vi "Auton_Selector.vi"(11 "Auton Name In":string) -> (3 "Auton Steps":T1[](array[typedef]))   [LabVIEW 2019]
uses:
  Drive/Drive Command Typedef.ctl
  Drive/Drive Mode Typedef.ctl
  Shoot/Shooter Command Type Def.ctl
  Shoot/Shooter Mode Type Def.ctl
  Intake/Intake Command Type Def.ctl
  Intake/Intake Mode Type Def.ctl
  <vilib>/Rock Robotics/WPI/Solenoid/WPI_SolenoidValue.ctl
  Auton Subsystems Steps Typedef.ctl
panel:
  in  "Possible autons":T9(array[cluster])
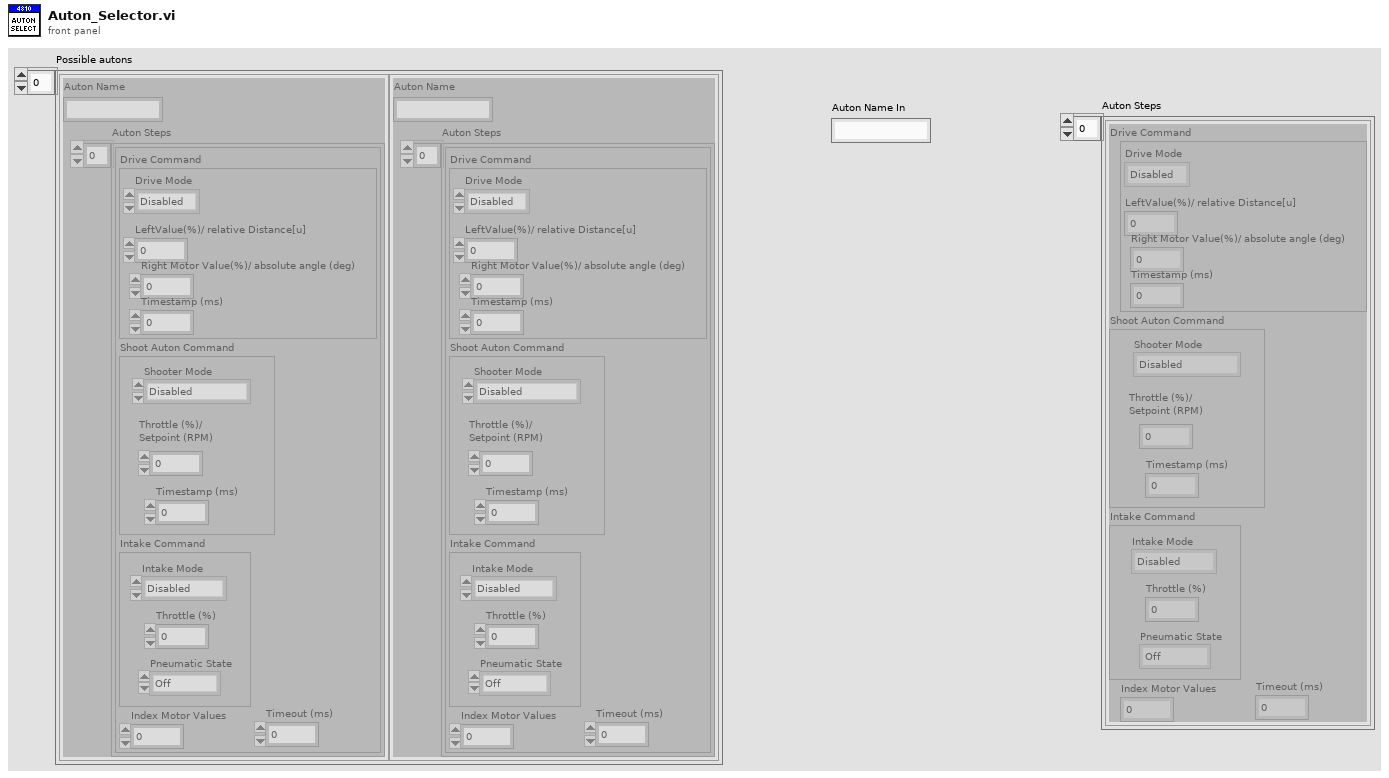
[diagram p1: front panel]
types:
  T1 = typedef "Auton Subsystems Steps Typedef.ctl" = cluster{"Drive Command":T2, "Shoot Auton Command":T4, "Intake Command":T6, "Index Motor Values":dbl, "Timeout (ms)":dbl}
  T2 = typedef "Drive Command Typedef.ctl" = cluster{"Drive Mode":T3, "LeftValue(%)/ relative Distance[u]":dbl, "Right Motor Value(%)/ absolute angle (deg)":dbl, "Timestamp (ms)":dbl}
  T3 = typedef "Drive Mode Typedef.ctl" = enum16{"Disabled", "Auto-align", "Drive Distance", "Turn to angle", "Driver"}
  T4 = typedef "Shooter Command Type Def.ctl" = cluster{"Shooter Mode":T5, "Throttle (%)/ \nSetpoint (RPM)":dbl, "Timestamp (ms)":dbl}
  T5 = typedef "Shooter Mode Type Def.ctl" = enum16{"Disabled", "Raw Throttle", "Velocity Control"}
  T6 = typedef "Intake Command Type Def.ctl" = cluster{"Intake Mode":T7, "Throttle (%)":dbl, "Pneumatic State":T8}
  T7 = typedef "Intake Mode Type Def.ctl" = enum16{"Disabled", "Enabled"}
  T8 = typedef "WPI_SolenoidValue.ctl" = enum16{"Off", "On", "Forward", "Reverse"}
  T9 = cluster{"Auton Name":string, "Auton Steps":T1[]}[]
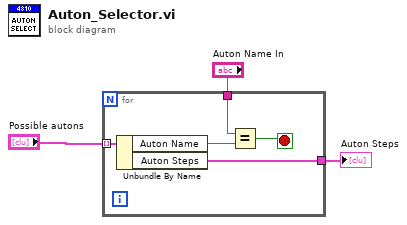
[diagram p0: block diagram]
diagram:
  n1 = for {
    tunnel: "Possible autons" -> [w8] mode=indexing
    tunnel: "Auton Name In" -> [w6]
    tunnel: [w4] -> w1
    stop <- w5 stop-if-true
    n2 = Unbundle By Name(w8) -> ("Auton Name"=w7:string, "Auton Steps"=w4:T1[])
    n3 = Equal?(x=w6, y=w7) -> (x = y?=w5:bool)
  }
  "Auton Steps" <- w1
